vi "_RIO Demo.vi"() -> ()   [LabVIEW 2012]
panel:
  in  "Go":bool
  in  "Script":string="SET Count,1\nloop:\nADD Count,1\nSET waittime,Count\nDIV waittime,5\nPRINT 0,Count\nPRINT 1,waittime\nDIO 4,1\nWAIT waittime\nDIO 4,0\nWAIT waittime\nIF (Count < 10) goto loop \nELSE  goto loop2\nloop2:"
  in  "stop":bool
  out "State":bool
  out "Btns":T1
  out "IP Address":string="Test"
  in  "LED":T2
  out "Waveform Chart":dbl(graph)
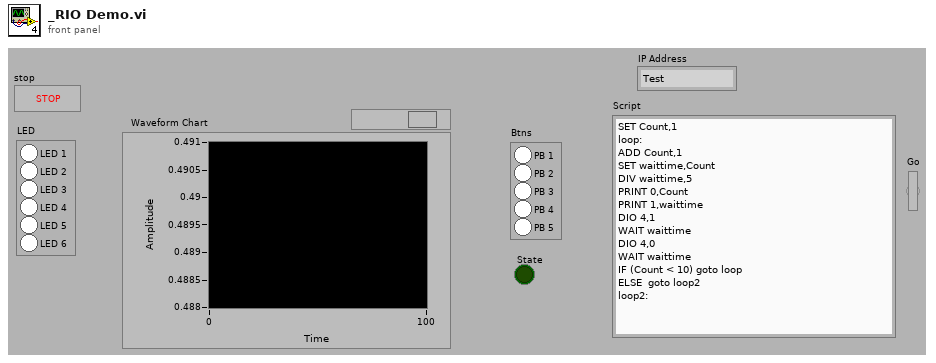
[diagram p1: front panel]
types:
  T1 = cluster{"PB 1":bool, "PB 2":bool, "PB 3":bool, "PB 4":bool, "PB 5":bool}
  T2 = cluster{"LED 1":bool, "LED 2":bool, "LED 3":bool, "LED 4":bool, "LED 5":bool, "LED 6":bool}
  T3 = typedef "RIO_Control.ctl" = cluster{"IP Address":string, "Connected?":bool, "connection ID":refnum<k5>, "Script":string}
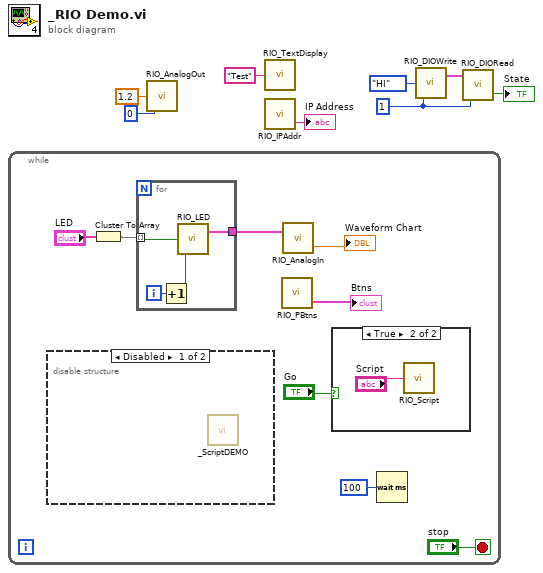
[diagram p0: block diagram]
diagram:
  w3 = u8 1 ("DIO Line")
  n1 = while {
    stop <- "stop" stop-if-true
    n2 = disable-structure shown="Disabled" {
      frame Disabled {
        n3 = call <userlib>:"_ScriptDEMO.vi"() -> ()  [unwired: 12 in]
      }
      frame Enabled {
      }
    }
    n4 = Cluster To Array(cluster="LED") -> (array=w13:bool[])
    n5 = for {
      tunnel: [w21] -> w12
      tunnel: w13 -> [w19] mode=indexing
      i -> [w20]
      n6 = Increment(x=w20) -> (x+1=w18:i32)
      n7 = call <userlib>:"RIO_LED.vi"("LED"=w18, "State"=w19) -> ("RIO Settings"=w21:T3)  [unwired: 2 in]
    }
    n8 = call <userlib>:"RIO_PBtns.vi"() -> ("Btns"=→"Btns":T1)  [unwired: 3 in, 1 out]
    n9 = call <userlib>:"RIO_AnalogIn.vi"("RIO Settings"=w12) -> ("voltage"=→"Waveform Chart":dbl)  [unwired: 1 in, 1 out]
    n10 = case shown="True" "Go" {
      frame False {
      }
      frame True {
        n11 = call <userlib>:"RIO_Script.vi"("Script"="Script") -> ()  [unwired: 3 in, 1 out]
      }
    }
    n12 = Wait (ms)(milliseconds to wait=u32 100) -> ()  [unwired: 1 out]
  }
  n13 = call <userlib>:"RIO_AnalogOut.vi"("DAC Channel"=u8 0, "voltage"=1.2) -> ()  [unwired: 2 in, 1 out]
  n14 = call <userlib>:"RIO_TextDisplay.vi"("Text"="Test") -> ()  [unwired: 3 in, 1 out]
  n15 = call <userlib>:"RIO_IPAddr.vi"() -> ("response"=→"IP Address":string)  [unwired: 3 in, 1 out]
  n16 = call <userlib>:"RIO_DIOWrite.vi"("DIO Line"=w3, "State"=enum16{"HI", "LO", "Toggle"}."HI") -> ("RIO Settings"=w2:T3)  [unwired: 2 in]
  n17 = call <userlib>:"RIO_DIORead.vi"("DIO Line"=w3, "RIO Settings"=w2) -> ("State"=→"State":bool)  [unwired: 1 in, 1 out]
